vi "Decide Action.vi"(8 "error in (no error)":errorcluster, 11 "MyMouse in":refnum<class "MyMouse.lvclass">) -> (0 "error out":errorcluster, 2 "Action":T1, 3 "MyMouse out":refnum<class "MyMouse.lvclass">)   [LabVIEW 2020, in "Mouse.lvlib" / "MyMouse.lvclass"]
uses:
  MyMouse.lvclass
  build/ppl/maze.lvlibp/Action.ctl
  build/ppl/maze.lvlibp/Mouse/Mouse.lvclass
  C:/dev/LabVIEW/Challenges/Maze/build/ppl/maze.lvlibp/Mouse/Mouse.lvclass
  build/ppl/maze.lvlibp
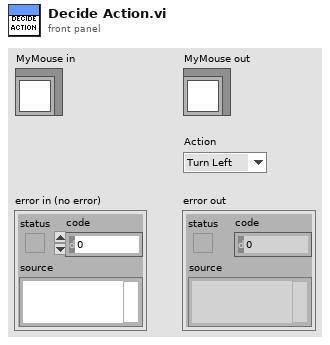
[diagram p1: front panel]
types:
  T1 = typedef "maze.lvlibp/Action.ctl" = enum16{"Turn Left", "Turn Right", "Forward"}
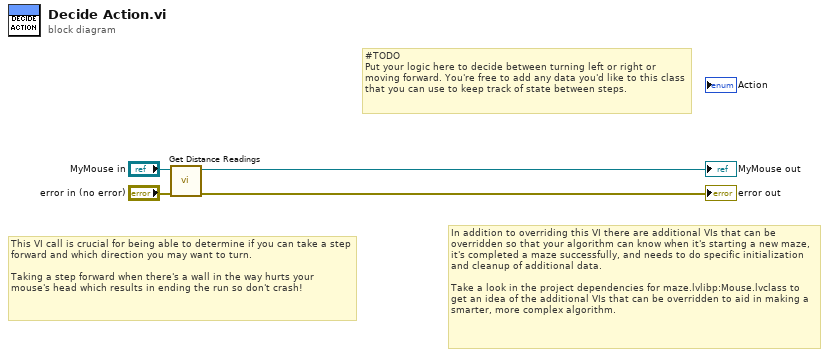
[diagram p0: block diagram]
diagram:
  # "In addition to overriding this VI there are additional VIs that can be overridden so that your algorithm can know when it's starting a new maze, it's completed a maze successfully, and needs to do specific initialization and cleanup of additional data.\n\nTake a look in the project dependencies for maze.lvlibp:Mouse.lvclass to get an idea of the additional VIs that can be overridden to aid in making a smarter, more complex algorithm."
  # "This VI call is crucial for being able to determine if you can take a step forward and which direction you may want to turn.\n\nTaking a step forward when there's a wall in the way hurts your mouse's head which results in ending the run so don't crash!"
  # "#TODO\nPut your logic here to decide between turning left or right or moving forward. You're free to add any data you'd like to this class that you can use to keep track of state between steps."
  n1 = call "Get Distance Readings.vi"("error in (no error)"="error in (no error)", "Mouse in"="MyMouse in") -> ("error out"=→"error out":errorcluster, "Mouse out"=→"MyMouse out":refnum<class "MyMouse.lvclass">)  [unwired: 7 in, 1 out]
